vi "Set Recording.vi"(8 "error in (no error)":errorcluster, 10 "Recording":bool, 11 "Dashboard Panel in":refnum<class "Dashboard Panel.lvclass">) -> (0 "error out":errorcluster, 3 "Dashboard Panel out":refnum<class "Dashboard Panel.lvclass">)   [LabVIEW 2020, in "SB App.lvlib" / "Dashboard Panel.lvclass"]
uses:
  Dashboard Panel.lvclass
  Dashboard Panel.lvclass/Dashboard Panel.ctl
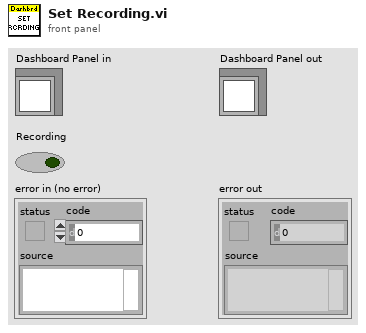
[diagram p1: front panel]
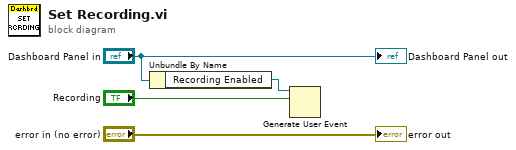
[diagram p0: block diagram]
diagram:
  n1 = Unbundle By Name("Dashboard Panel in") -> ("Recording Enabled"=w3:refnum<user-event>)
  n2 = Generate User Event(user event=w3, event data cluster="Recording") -> ()  [unwired: 2 in, 2 out]
  "error out" <- "error in (no error)"
  "Dashboard Panel out" <- "Dashboard Panel in"
